vi "ImageFrame.vi"(0 "Tasks In":T2, 1 "Vphases":dbl[](array[numeric]), 5 "Global Parameters":T1={"DC AI Min (V)"=0.0015, "DC AI Max (V)"=0.06, "Mixer AI Min (V)"=-0.3, "Mixer AI Max (V)"=0.3, "Bias AO Min (V)"=-1.0, "Bias AO Max (V)"=7.0, "Scan AO Min (V)"=-10.0, "Scan AO Max (V)"=10.0, "Fast Samp Freq (Hz)"=2500000.0, "Slow Samp Freq (Hz)"=250000.0}, 7 "Calibration Parameters":T4={"Target Lifetime (s)"=4e-09, "Integration Time (s)"=0.1, "Calibration Steps"=500.0}, 9 "Functions":T3(ring)=enum."Measurement", 11 "error in":errorcluster, 12 "index":dbl, 13 "XYcoordinates":dbl[][](array[numeric])) -> (4 "Tasks Out":T2, 6 "Mixer AI Channels Data":dbl[][](array[numeric]) format="%0.2f", 8 "DC AI Channel Date":dbl[](array[numeric]) format="%0.2f", 10 "Bias Voltage":dbl, 15 "error out":errorcluster)   [LabVIEW 2015]
uses:
  <vilib>/DAQmx/write.llb/DAQmx Write (Analog 1D DBL NChan 1Samp).vi
  <vilib>/DAQmx/write.llb/DAQmx Write (Analog 2D DBL NChan NSamp).vi
  <vilib>/DAQmx/read.llb/DAQmx Read (Analog 2D DBL NChan NSamp).vi
  <vilib>/DAQmx/read.llb/DAQmx Read (Analog 1D DBL 1Chan NSamp).vi
  <vilib>/DAQmx/miscellaneous.llb/DAQmx Fill In Error Info.vi
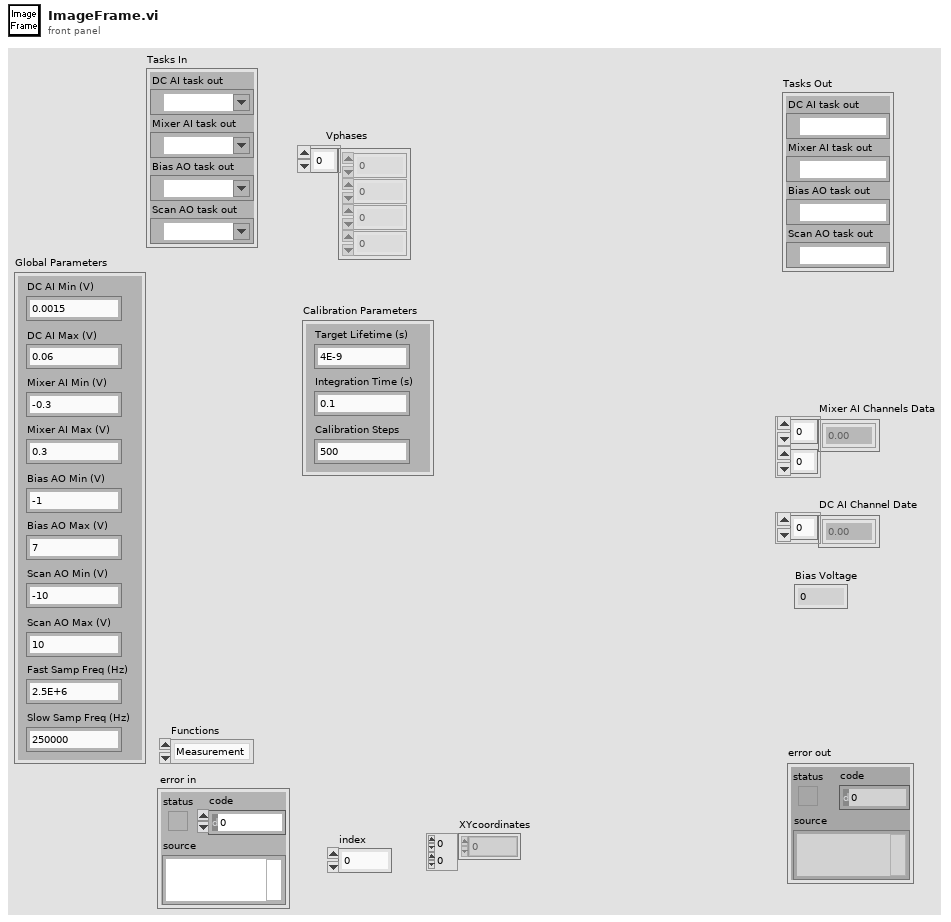
[diagram p1: front panel]
types:
  T1 = cluster{"DC AI Min (V)":dbl, "DC AI Max (V)":dbl, "Mixer AI Min (V)":dbl, "Mixer AI Max (V)":dbl, "Bias AO Min (V)":dbl, "Bias AO Max (V)":dbl, "Scan AO Min (V)":dbl, "Scan AO Max (V)":dbl, "Fast Samp Freq (Hz)":dbl, "Slow Samp Freq (Hz)":dbl}
  T2 = cluster{"DC AI task out":refnum<k21>, "Mixer AI task out":refnum<k21>, "Bias AO task out":refnum<k21>, "Scan AO task out":refnum<k21>}
  T3 = enum32{"Calibration", "Fast Scan", "Measurement"}
  T4 = cluster{"Target Lifetime (s)":dbl, "Integration Time (s)":dbl, "Calibration Steps":dbl}
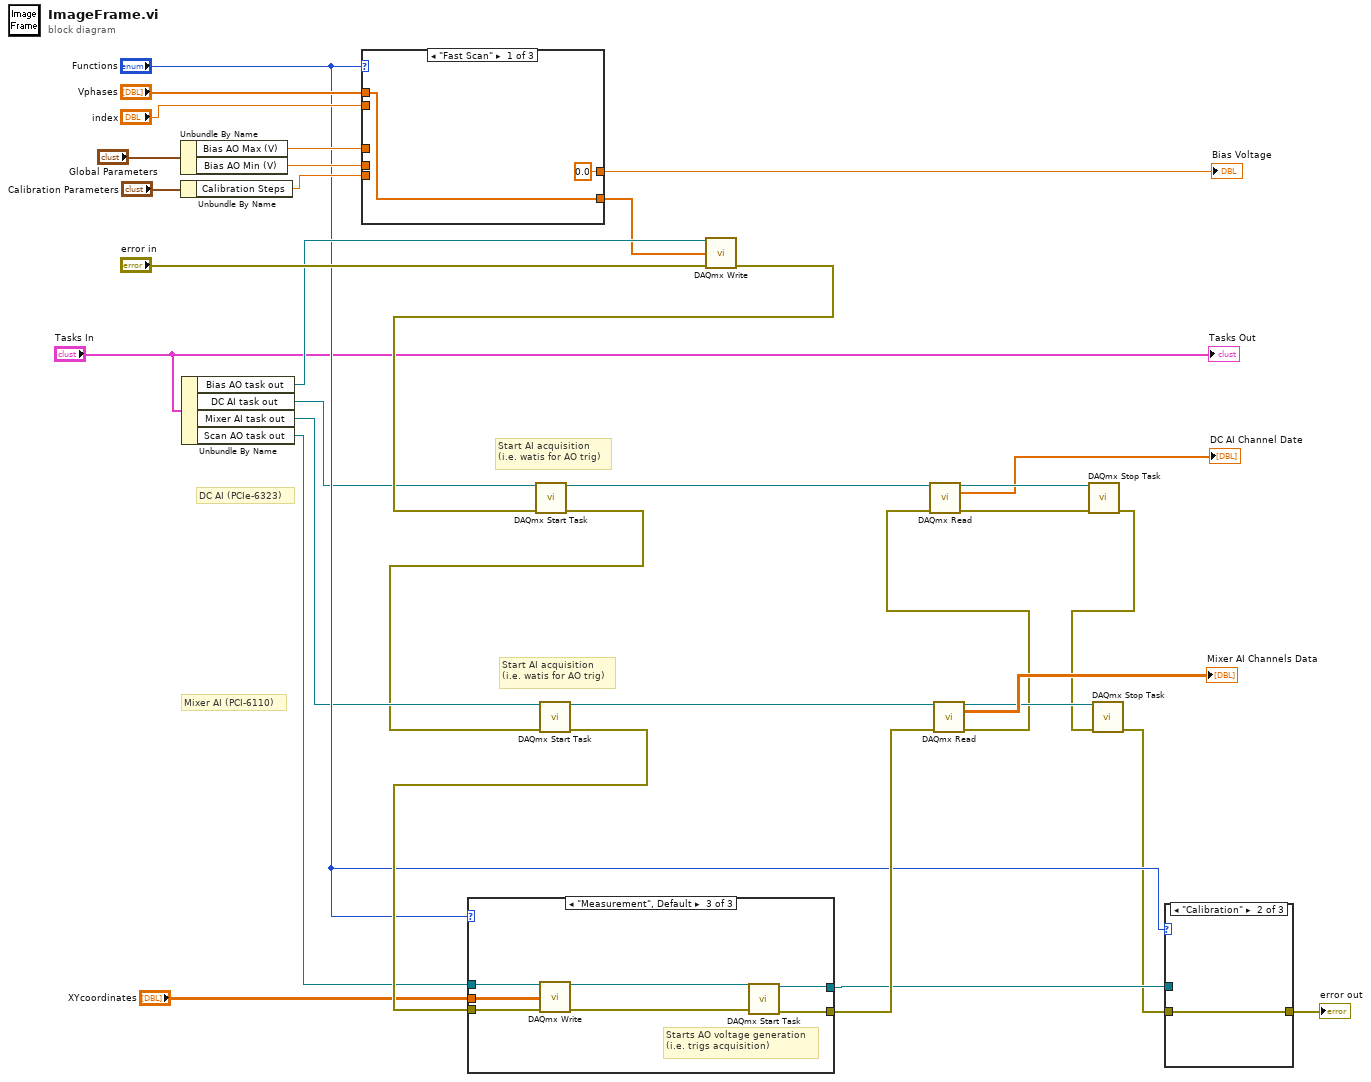
[diagram p0: block diagram]
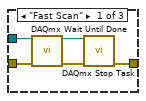
[diagram p2: hidden frame]
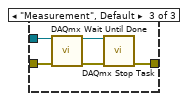
[diagram p3: hidden frame]
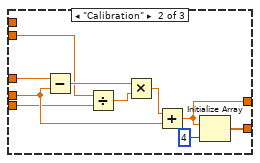
[diagram p4: hidden frame]
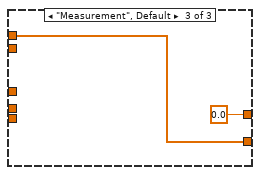
[diagram p5: hidden frame]
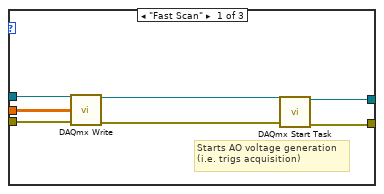
[diagram p6: hidden frame]
diagram:
  # "Start AI acquisition\n(i.e. watis for AO trig)"
  # "DC AI (PCIe-6323)"
  # "Mixer AI (PCI-6110)"
  # "Start AI acquisition\n(i.e. watis for AO trig)"
  n1 = Unbundle By Name("Global Parameters") -> ("Bias AO Max (V)"=w29:dbl, "Bias AO Min (V)"=w28:dbl)
  n2 = Unbundle By Name("Calibration Parameters") -> ("Calibration Steps"=w27:dbl)
  n3 = Unbundle By Name("Tasks In") -> ("Bias AO task out"=w25:refnum<k21>, "DC AI task out"=w3:refnum<k21>, "Mixer AI task out"=w12:refnum<k21>, "Scan AO task out"=w13:refnum<k21>)
  n4 = case shown="\"Fast Scan\"" "Functions" {
    tunnel: "Vphases" -> [w34 _ w47]
    tunnel: "index" -> [_ w42 _]
    tunnel: w29 -> [_ w41 _]
    tunnel: w28 -> [_ w40 _]
    tunnel: w27 -> [_ w39 _]
    tunnel: [w34 w37 w47] -> w14
    tunnel: [0.0 w36 0.0] -> w15
    frame "Fast Scan" {
    }
    frame "Calibration" {
      n5 = Subtract(x=w41, y=w40) -> (x-y=w45:dbl)
      n6 = Divide(x=w42, y=w39) -> (x/y=w44:dbl)
      n7 = Multiply(x=w45, y=w44) -> (x*y=w43:dbl)
      n8 = Add(x=w43, y=w40) -> (x+y=w36:dbl)
      n9 = Initialize Array(w36, 4 ("dimension size")) -> (w37:dbl[])
    }
    frame "Measurement", Default {
    }
  }
  "Bias Voltage" <- w15
  n10 = call-poly <vilib>:"DAQmx Write.vi"("task/channels in"=w25, "data"=w14, "error in"="error in") -> ("error out"=w7:errorcluster)  [unwired: 10 in, 2 out]
  n11 = call <vilib>:"DAQmx Start Task.vi"("task/channels in"=w3, "error in"=w7) -> ("task out"=w8:refnum<k21>, "error out"=w6:errorcluster)  [unwired: 12 in]
  n12 = call <vilib>:"DAQmx Start Task.vi"("task/channels in"=w12, "error in"=w6) -> ("task out"=w33:refnum<k21>, "error out"=w24:errorcluster)  [unwired: 12 in]
  n13 = case shown="\"Measurement\", Default" "Functions" {
    tunnel: w24 -> [w49 w55 w61]
    tunnel: w13 -> [w50 w56 w60]
    tunnel: "XYcoordinates" -> [w48 _ w59]
    tunnel: [w52 w56 w58] -> w20
    tunnel: [w51 w55 w57] -> w22
    frame "Fast Scan" {
      # "Starts AO voltage generation\n(i.e. trigs acquisition)"
      n14 = call-poly <vilib>:"DAQmx Write.vi"("task/channels in"=w50, "data"=w48, "error in"=w49) -> ("task out"=w53:refnum<k21>, "error out"=w54:errorcluster)  [unwired: 10 in, 1 out]
      n15 = call <vilib>:"DAQmx Start Task.vi"("task/channels in"=w53, "error in"=w54) -> ("task out"=w52:refnum<k21>, "error out"=w51:errorcluster)  [unwired: 12 in]
    }
    frame "Calibration" {
    }
    frame "Measurement", Default {
      # "Starts AO voltage generation\n(i.e. trigs acquisition)"
      n16 = call-poly <vilib>:"DAQmx Write.vi"("task/channels in"=w60, "data"=w59, "error in"=w61) -> ("task out"=w62:refnum<k21>, "error out"=w63:errorcluster)  [unwired: 10 in, 1 out]
      n17 = call <vilib>:"DAQmx Start Task.vi"("task/channels in"=w62, "error in"=w63) -> ("task out"=w58:refnum<k21>, "error out"=w57:errorcluster)  [unwired: 12 in]
    }
  }
  n18 = call-poly <vilib>:"DAQmx Read.vi"("task/channels in"=w33, "error in"=w22) -> ("task out"=w16:refnum<k21>, "data"=→"Mixer AI Channels Data":dbl[][], "error out"=w5:errorcluster)  [unwired: 11 in]
  n19 = call-poly <vilib>:"DAQmx Read.vi"("task/channels in"=w8, "error in"=w5) -> ("task out"=w10:refnum<k21>, "data"=→"DC AI Channel Date":dbl[], "error out"=w11:errorcluster)  [unwired: 11 in]
  n20 = call <vilib>:"DAQmx Stop Task.vi"("task/channels in"=w10, "error in"=w11) -> ("error out"=w4:errorcluster)  [unwired: 12 in, 1 out]
  n21 = call <vilib>:"DAQmx Stop Task.vi"("task/channels in"=w16, "error in"=w4) -> ("error out"=w19:errorcluster)  [unwired: 12 in, 1 out]
  n22 = case shown="\"Calibration\"" "Functions" {
    tunnel: w20 -> [w66 _ w72]
    tunnel: w19 -> [w65 w69 w71]
    tunnel: [w64 w69 w70] -> w18
    frame "Fast Scan" {
      n23 = call <vilib>:"DAQmx Wait Until Done.vi"("task/channels in"=w66, "error in"=w65) -> ("task out"=w68:refnum<k21>, "error out"=w67:errorcluster)  [unwired: 12 in]
      n24 = call <vilib>:"DAQmx Stop Task.vi"("task/channels in"=w68, "error in"=w67) -> ("error out"=w64:errorcluster)  [unwired: 12 in, 1 out]
    }
    frame "Calibration" {
    }
    frame "Measurement", Default {
      n25 = call <vilib>:"DAQmx Wait Until Done.vi"("task/channels in"=w72, "error in"=w71) -> ("task out"=w73:refnum<k21>, "error out"=w74:errorcluster)  [unwired: 12 in]
      n26 = call <vilib>:"DAQmx Stop Task.vi"("task/channels in"=w73, "error in"=w74) -> ("error out"=w70:errorcluster)  [unwired: 12 in, 1 out]
    }
  }
  "error out" <- w18
  "Tasks Out" <- "Tasks In"
